vi "Is Dynamic Dispatch.vi"(8 "error in (no error)":errorcluster, 11 "Data in":T1) -> (0 "error out":errorcluster, 2 "Is Dynamic Dispatch?":bool, 3 "Data out":T1)   [LabVIEW 2020, in "Peek Window.lvlib"]
uses:
  Peek Window.lvlib
  MHL Data Cluster.ctl
  Open Diagram Argument--cluster.ctl
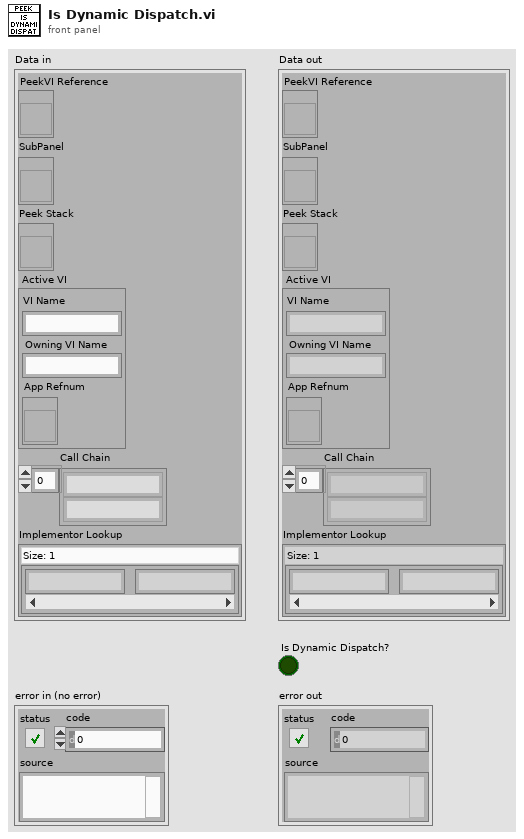
[diagram p1: front panel]
types:
  T1 = typedef "Peek Window.lvlib/MHL Data Cluster.ctl" = cluster{"PeekVI Reference":refnum<vi>, "SubPanel":refnum<vi>, "Peek Stack":refnum<vi>, "Active VI":T2, "Call Chain":string[], "Implementor Lookup":map{string, string}}
  T2 = typedef "Peek Window.lvlib/Open Diagram Argument--cluster.ctl" = cluster{"VI Name":string, "Owning VI Name":string, "App Refnum":refnum<vi>}
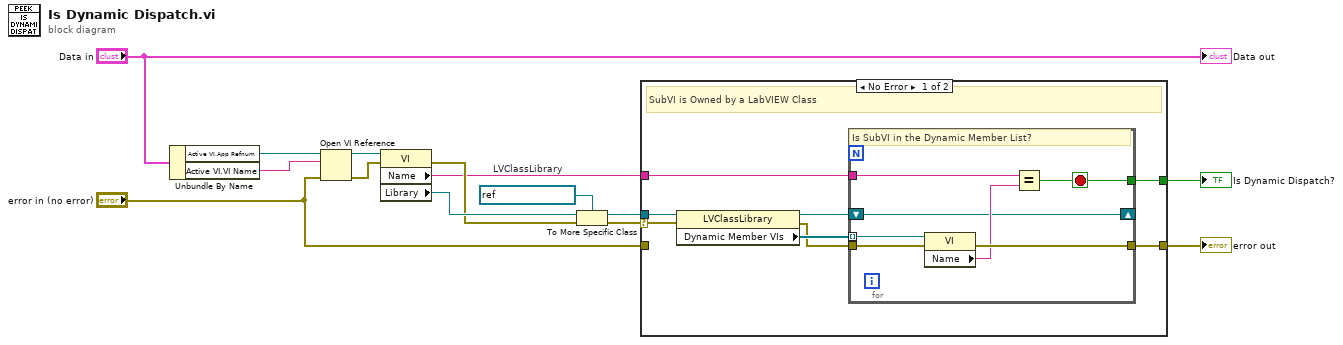
[diagram p0: block diagram]
diagram:
  w14 = refnum<vi> refnum  # LVClassLibrary
  n1 = Unbundle By Name("Data in") -> ("Active VI.App Refnum"=w7:refnum<vi>, "Active VI.VI Name"=w6:string)
  n2 = Open VI Reference(application reference (local)=w7, vi path=w6, error in (no error)="error in (no error)") -> (vi reference=w5:refnum<vi>, error out=w4:errorcluster)  [unwired: 3 in]
  n3 = property class="VI"(reference=w5, error in=w4) -> (error out=w9:errorcluster, "Name"=w3:string, "Library"=w10:refnum<vi>)  [unwired: 1 out]
  n4 = To More Specific Class(target class=w14, reference=w10, error in=w9) -> (specific class reference=w13:refnum<vi>, error out=w12:errorcluster)
  n5 = case shown="No Error" w12 {
    selector: w12 -> [w21 _]
    tunnel: w13 -> [w22 _]
    tunnel: w3 -> [w20 _]
    tunnel: [w16 _] -> w11
    tunnel: [w15 w30] -> w2
    tunnel: "error in (no error)" -> [_ w30]
    frame No Error {
      # "SubVI is Owned by a LabVIEW Class"
      n6 = property class="LVClassLibrary"(reference=w22, error in=w21) -> (reference out=w17:refnum<vi>, error out=w18:errorcluster, "Dynamic Member VIs"=w19:refnum<vi>[])
      n7 = for {
        tunnel: w20 -> [w28]
        tunnel: w19 -> [w29] mode=indexing
        tunnel: w18 -> [w27]
        tunnel: [w26] -> w15
        tunnel: [w25] -> w16
        shift-right: [w23] -> _
        shift-left: w17 -> [w23]
        stop <- w25 stop-if-true
        # "Is SubVI in the Dynamic Member List?"
        n8 = property class="VI"(reference=w29, error in=w27) -> (error out=w26:errorcluster, "Name"=w24:string)  [unwired: 1 out]
        n9 = Equal?(x=w28, y=w24) -> (x = y?=w25:bool)
      }
    }
    frame Error {
      # "Not in a Class or in a Library"
    }
  }
  "error out" <- w2
  "Is Dynamic Dispatch?" <- w11
  "Data out" <- "Data in"
